vi "XML Config.vi"(10 "indent levels":i32, 11 "Controls in":refnum<vi>[](array[refnum])) -> (3 "XML":string)   [LabVIEW 2013, in "XML Config.lvlib"]
uses:
  XML Config.lvlib
panel:
  out "size(s)":i32
  out "Number of Columns":u32
  out "error out":errorcluster
  out "Number of Rows":u32
  out "Label":string[](array[string])
  out "Class name":string[](array[string])
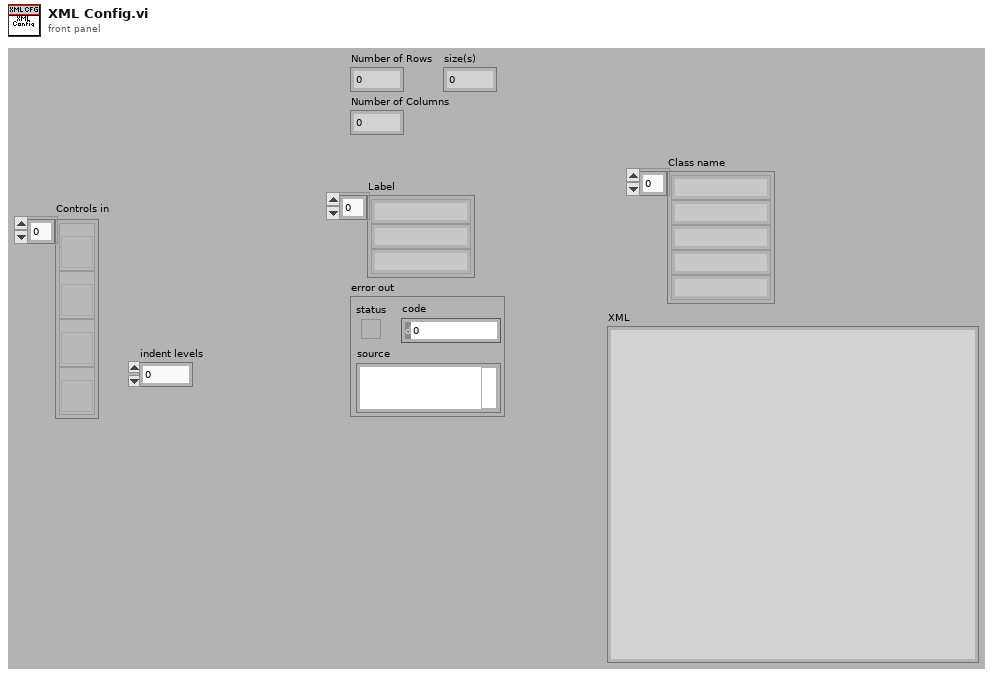
[diagram p1: front panel]
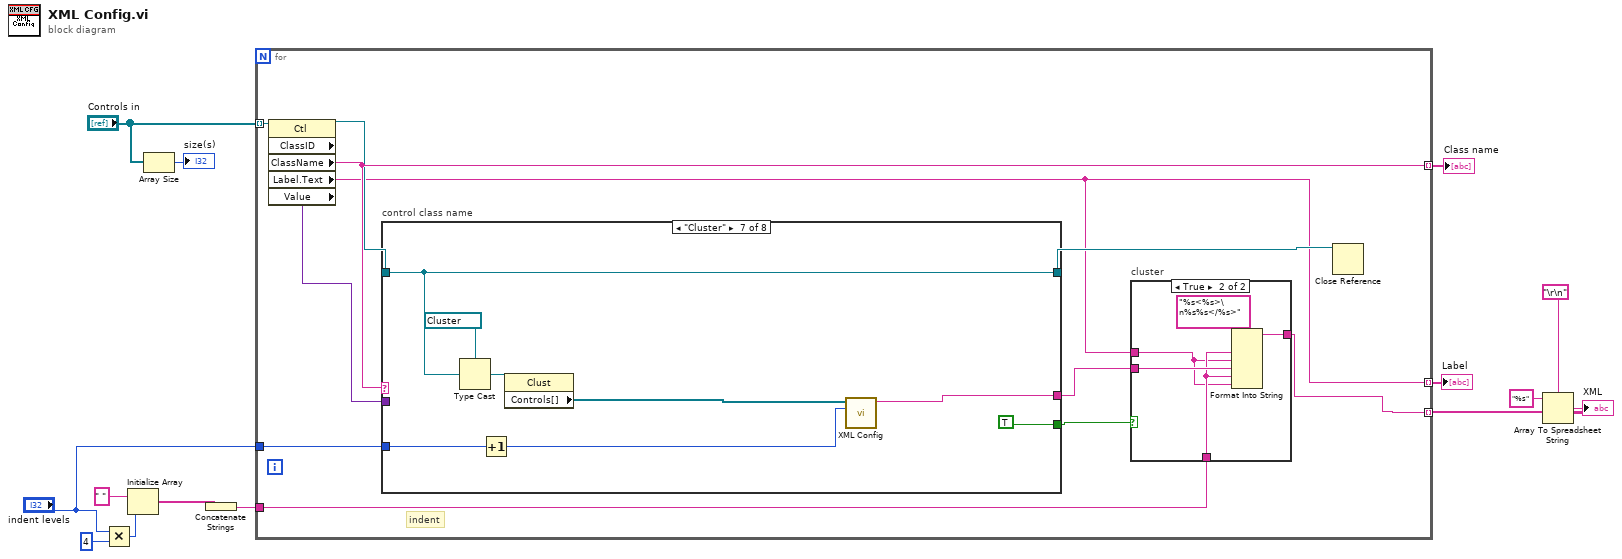
[diagram p0: block diagram]
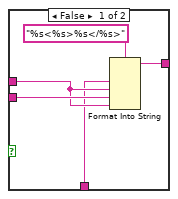
[diagram p2: hidden frame]
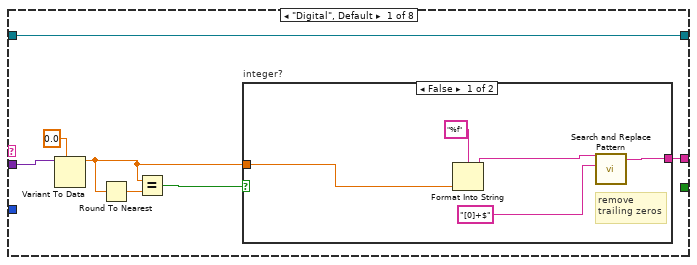
[diagram p3: hidden frame]
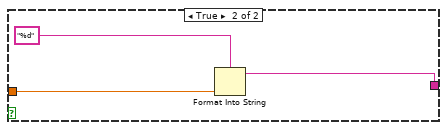
[diagram p4: hidden frame]
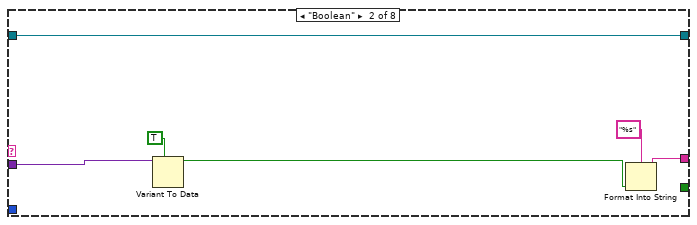
[diagram p5: hidden frame]
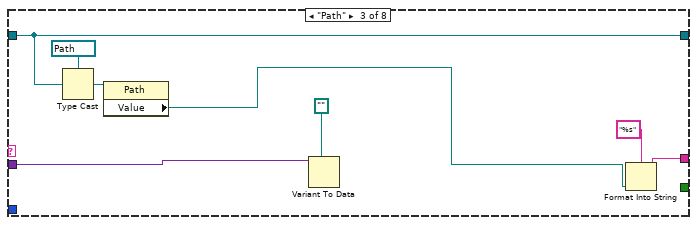
[diagram p6: hidden frame]
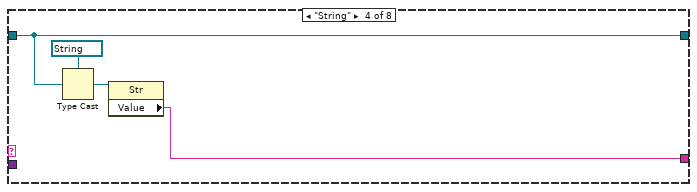
[diagram p7: hidden frame]
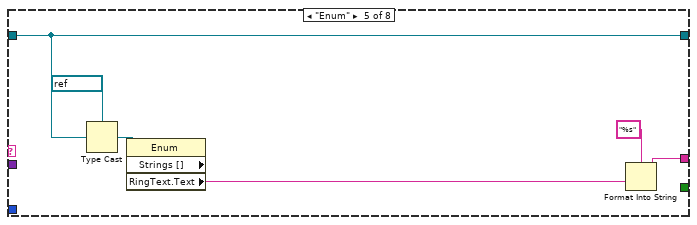
[diagram p8: hidden frame]
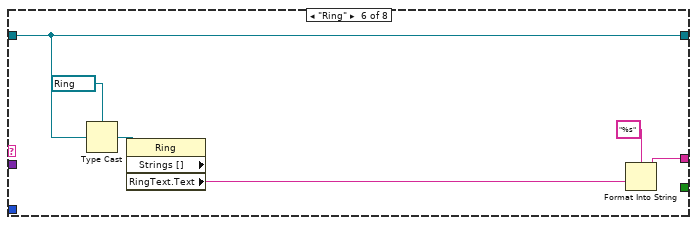
[diagram p9: hidden frame]
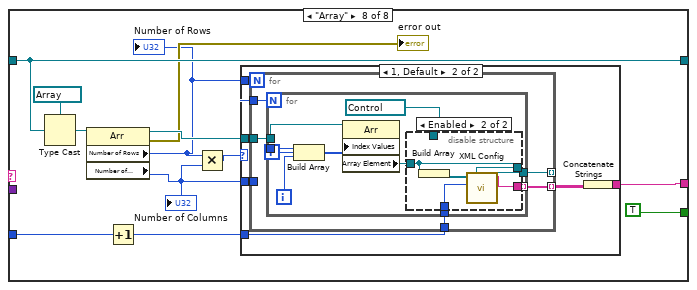
[diagram p10: hidden frame]
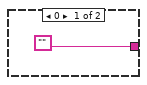
[diagram p11: hidden frame]
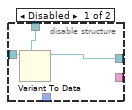
[diagram p12: hidden frame]
diagram:
  n1 = Multiply(x="indent levels", y=4) -> (x*y=w3:i32)
  n2 = Initialize Array(" " ("format string"), w3) -> (w7:string[])
  n3 = Array Size(array="Controls in") -> (size(s)=→"size(s)":i32)
  n4 = Concatenate Strings(w7) -> (w6:string)
  n5 = for {
    tunnel: [w25] -> w14 mode=indexing
    tunnel: [w18] -> w13 mode=indexing
    tunnel: [w21] -> w9 mode=indexing
    tunnel: "Controls in" -> [w19] mode=indexing
    tunnel: w6 -> [w17]
    tunnel: "indent levels" -> [w16]
    # "indent"
    n6 = property class="Ctl" props=["ClassID", "ClassName", "Label", "Text", "Value"](reference=w19) -> (reference out=w23:refnum<vi>, "ClassName"=w25:string, "Label.Text"=w18:string, "Value"=w24:variant)  [unwired: 1 in, 2 out]
    n7 = case "control class name" shown="\"Cluster\"" w25 {
      tunnel: w24 -> [w42 w56 w64 _ _ _ _ _]
      tunnel: [w40 w53 w62 w65 w73 w79 w82 w93] -> w20
      tunnel: w23 -> [w36 w51 w58 w66 w69 w75 w86 w99]
      tunnel: [w36 w51 w58 w66 w69 w75 w86 w99] -> w22
      tunnel: w16 -> [_ _ _ _ _ _ w84 w98]
      tunnel: [_ _ _ _ _ _ TRUE TRUE] -> w15
      frame "Digital", Default {
        n8 = Variant To Data(type=0.0, Variant=w42) -> (data=w39:dbl)  [unwired: 1 in, 1 out]
        n9 = Round To Nearest(number=w39) -> (nearest integer value=w38:dbl)
        n10 = Equal?(x=w39, y=w38) -> (x = y?=w37:bool)
        n11 = case "integer?" shown="False" w37 {
          tunnel: [w43 w48] -> w40
          tunnel: w39 -> [w46 w50]
          frame False {
            # "remove\ntrailing zeros"
            n12 = Format Into String(format string="%f", w46) -> (resulting string=w44:string)  [unwired: 2 in, 1 out]
            n13 = call <vilib>:"Search and Replace Pattern.vi"("string"=w44, "regular expression (\"\")"="[0]+$" ("regular expression (\"\")")) -> ("result string"=w43:string)  [unwired: 3 in, 1 out]
          }
          frame True {
            n14 = Format Into String(format string="%d", w50) -> (resulting string=w48:string)  [unwired: 2 in, 1 out]
          }
        }
      }
      frame "Boolean" {
        n15 = Variant To Data(type=TRUE, Variant=w56) -> (data=w54:bool)  [unwired: 1 in, 1 out]
        n16 = Format Into String(format string="%s", w54) -> (resulting string=w53:string)  [unwired: 2 in, 1 out]
      }
      frame "Path" {
        n17 = Type Cast(type=refnum<vi> refnum ("Enum"), x=w58) -> (*(type *) &x=w59:refnum<vi>)
        n18 = property class="Path"(reference=w59) -> ("Value"=w57:path)  [unwired: 1 in, 2 out]
        n19 = Variant To Data(type=path "", Variant=w64) -> ()  [unwired: 1 in, 2 out]
        n20 = Format Into String(format string="%s", w57) -> (resulting string=w62:string)  [unwired: 2 in, 1 out]
      }
      frame "String" {
        n21 = Type Cast(type=refnum<vi> refnum ("Enum"), x=w66) -> (*(type *) &x=w67:refnum<vi>)
        n22 = property class="Str"(reference=w67) -> ("Value"=w65:string)  [unwired: 1 in, 2 out]
      }
      frame "Enum" {
        n23 = Type Cast(type=refnum<vi> refnum ("Enum"), x=w69) -> (*(type *) &x=w71:refnum<vi>)
        n24 = property class="Enum" props=["Strings []", "RingText", "Text"](reference=w71) -> ("RingText.Text"=w70:string)  [unwired: 1 in, 3 out]
        n25 = Format Into String(format string="%s", w70) -> (resulting string=w73:string)  [unwired: 2 in, 1 out]
      }
      frame "Ring" {
        n26 = Type Cast(type=refnum<vi> refnum ("Enum"), x=w75) -> (*(type *) &x=w77:refnum<vi>)
        n27 = property class="Ring" props=["Strings []", "RingText", "Text"](reference=w77) -> ("RingText.Text"=w76:string)  [unwired: 1 in, 3 out]
        n28 = Format Into String(format string="%s", w76) -> (resulting string=w79:string)  [unwired: 2 in, 1 out]
      }
      frame "Cluster" {
        n29 = Type Cast(type=refnum<vi> refnum ("Enum"), x=w86) -> (*(type *) &x=w87:refnum<vi>)
        n30 = Increment(x=w84) -> (x+1=w83:i32)
        n31 = property class="Clust"(reference=w87) -> ("Controls[]"=w85:refnum<vi>[])  [unwired: 1 in, 2 out]
        n32 = call "XML Config.vi"("indent levels"=w83, "Controls in"=w85) -> ("XML"=w82:string)  [unwired: 9 in]
      }
      frame "Array" {
        n33 = Type Cast(type=refnum<vi> refnum ("Enum"), x=w99) -> (*(type *) &x=w96:refnum<vi>)
        n34 = property class="Arr"(reference=w96) -> (reference out=w95:refnum<vi>, error out=→"error out":errorcluster, "Number of Rows"=w91:u32, "Number of Columns"=w90:u32)  [unwired: 1 in]
        "Number of Rows" <- w91
        "Number of Columns" <- w90
        n35 = Increment(x=w98) -> (x+1=w92:i32)
        n36 = Multiply(x=w91, y=w90) -> (x*y=w89:u32)
        n37 = case shown="1, Default" w89 {
          tunnel: w95 -> [_ w107]
          tunnel: ["" w105] -> w93
          tunnel: w92 -> [_ w104]
          tunnel: w91 -> [_ w103]
          tunnel: w90 -> [_ w102]
          frame 0 {
          }
          frame 1, Default {
            n38 = for {
              N: w103 -> [_]
              tunnel: w107 -> [w113]
              tunnel: w102 -> [_]
              tunnel: [w112] -> _ mode=indexing
              tunnel: w102 -> [w110]
              tunnel: [w109] -> w106 mode=indexing
              tunnel: w104 -> [w108]
              i -> [w111]
              n39 = for {
                N: w110 -> [_]
                tunnel: w113 -> [w122]
                tunnel: [w120] -> w112
                tunnel: w111 -> [w119]
                tunnel: [w115] -> w109 mode=indexing
                tunnel: w108 -> [w114]
                i -> [w116]
                n40 = Build Array(w119, w116) -> (w118:i32[])
                n41 = property class="Arr"(reference=w122, "Index Values"=w118) -> ("Array Element"=w117:refnum<vi>)  [unwired: 1 in, 2 out]
                n42 = disable-structure shown="Enabled" {
                  disable-tunnel: refnum<vi> refnum ("Enum") -> [w125 _]
                  disable-tunnel: [w124 w129] -> w120
                  disable-tunnel: w117 -> [w123 w129]
                  disable-tunnel: [_ w127] -> w115
                  disable-tunnel: w114 -> [_ w126]
                  frame Disabled {
                    n43 = Variant To Data(type=w125, Variant=w123) -> (data=w124:refnum<vi>)  [unwired: 1 in, 1 out]
                  }
                  frame Enabled {
                    n44 = Build Array(w129) -> (w128:refnum<vi>[])
                    n45 = call "XML Config.vi"("indent levels"=w126, "Controls in"=w128) -> ("XML"=w127:string)  [unwired: 9 in]
                  }
                }
              }
            }
            n46 = Concatenate Strings(w106) -> (w105:string)
          }
        }
      }
    }
    n47 = case "cluster" shown="True" w15 {
      tunnel: [w29 w34] -> w21
      tunnel: w20 -> [w28 w33]
      tunnel: w18 -> [w27 w31]
      tunnel: w17 -> [w26 w32]
      frame False {
        n48 = Format Into String(format string="%s<%s>%s</%s>", w26, w27, w28, w27) -> (resulting string=w29:string)  [unwired: 2 in, 1 out]
      }
      frame True {
        n49 = Format Into String(format string="%s<%s>\n%s%s</%s>", w32, w31, w33, w32, w31) -> (resulting string=w34:string)  [unwired: 2 in, 1 out]
      }
    }
    n50 = Close Reference(reference=w22) -> ()  [unwired: 1 in, 1 out]
  }
  "Class name" <- w14
  "Label" <- w13
  n51 = Array To Spreadsheet String(delimiter (Tab)="\r\n", array=w9, 3:"%s" ("format string")) -> (spreadsheet string=→"XML":string)
